vi "OE1022_Configure DAC.vi"(7 "OE1022_Configure DAC":T1 {"DAC4 Output" min=-10.0 max=10.0 format="%#_4g"; "DAC3 Output" min=-10.0 max=10.0 format="%#_4g"; "DAC2 Output" min=-10.0 max=10.0 format="%#_4g"; "DAC1 Output" min=-10.0 max=10.0 format="%#_4g"}, 8 "Error in (no error)":errorcluster caption="error out（no error）", 9 "Remote Mode":u16(ring) items=["USB"=0, "GPIB"=2], 11 "VISA resource name":refnum<visa-resource-name>) -> (0 "Error out":errorcluster caption="error out", 1 "Output String":string, 3 "VISA resource  out":refnum<visa-resource-name>)   [LabVIEW 2011]
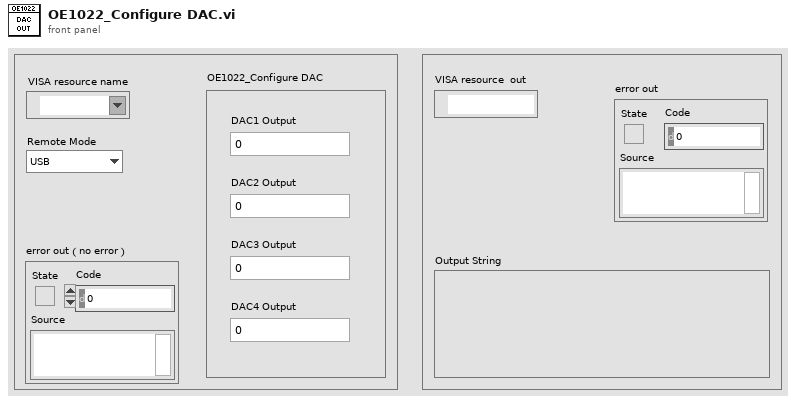
[diagram p1: front panel]
types:
  T1 = cluster{"DAC1 Output":dbl, "DAC2 Output":dbl, "DAC3 Output":dbl, "DAC4 Output":dbl}
  T2 = enum16{"ISRC", "IGND", "ICPL", "ILIN", "PHAS", "FMOD", "RSLP", "FREQ", "SWPT", "SLLM", "SULM", "SSLL", "SSLG", "STLM", "SWRM", "IRNG", "SENS", "RMOD", "OFLT", "OFSL", "SYNC", "DMOD", "HARM", "DARB", "SWVT", "SLVL", "SVLL", "SVUL", "SVSL", "SVSG", "SVTM", "SVRM", "RALL", "SNAP", "OUTP", "OAUX", "COUT", "CAUX", "COFP", "CEXP", "FPOP", "OEXP", "*IDN", "*RST", "OVLD", "INOV", "GNOV", "*PLL", "SSET", "RSET", "AGAN", "APHS", "ARSV", "ASCL", "EQCD", "EQCS", "SPED", "SRAT", "SLEN", "SSLE", "STRG", "SPRM", "STRD", "PAUS", "REST", "SPTS", "TRCA", "TEMP", "RSTU", "IHNZ", "DEQU", "SADD", "ARNG", "CSPE", "ISRCD", "IGNDD", "ICPLD", "ILIND", "PHASD", "FMODD", "RSLPD", "FREQD", "SWPTD", "SLLMD", "SULMD", "SSLLD", "SSLGD", "STLMD", "SWRMD", "SENSD", "RMODD", "OFLTD", "OFSLD", "SYNCD", "HARMD", "EQCDD", "EQCSD", "SNAPD", "OUTPD", "SWVTD", "SLVLD", "SVLLD", "SVULD", "SVSLD", "SVSGD", "SVTMD", "SVRMD", "SVDCD", "ARSVD", "AGAND", "APHSD", "ASCLD", "FPOPD", "CAUXD", "OEXPD", "SPEDD", "SRATD", "SLEND", "SSLED", "STRGD", "SPRMD", "STRDD", "PAUSD", "RESTD", "SPTSD", "TRCAD", "*IDND", "*RSTD", "INOVD", "GNOVD", "*PLLD", "SSETD", "RSETD"}
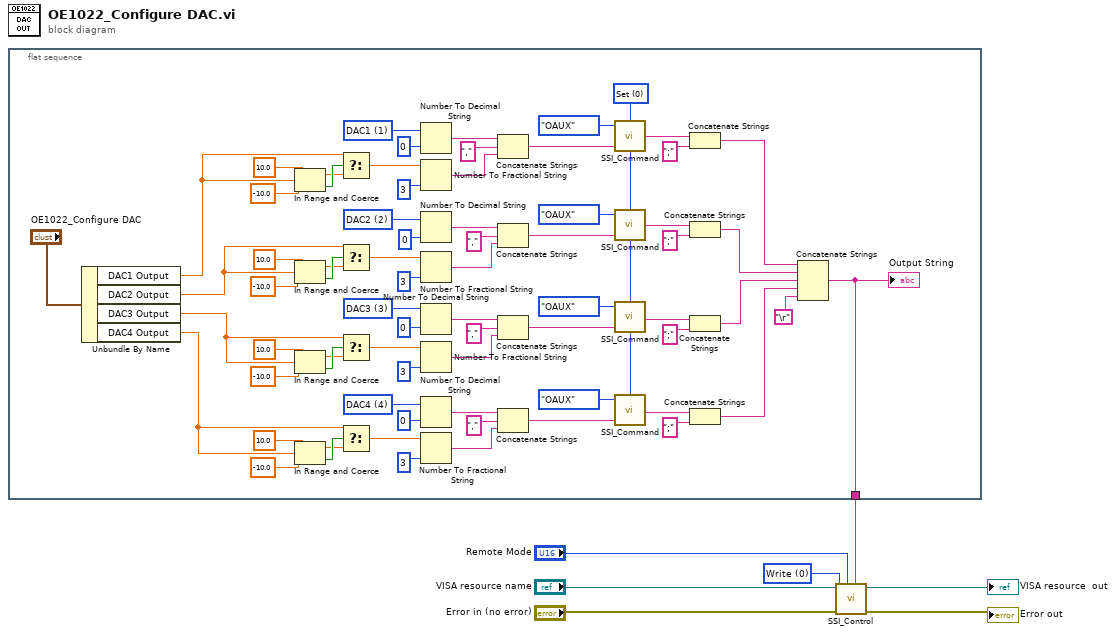
[diagram p0: block diagram]
diagram:
  w6 = u16 0 items=["Write", "Read"] ("Control")
  n1 = flat-sequence {
    tunnel: [w70] -> w1
    frame #0 {
      w8 = u16 0 items=["Set", "Query"] ("Opera")
      w9 = u16 4 items=["DAC1"=1, "DAC2"=2, "DAC3"=3, "DAC4"=4]
      w10 = u16 3 items=["DAC1"=1, "DAC2"=2, "DAC3"=3, "DAC4"=4]
      w11 = u16 2 items=["DAC1"=1, "DAC2"=2, "DAC3"=3, "DAC4"=4]
      w12 = u16 1 items=["DAC1"=1, "DAC2"=2, "DAC3"=3, "DAC4"=4]
      n2 = Unbundle By Name("OE1022_Configure DAC") -> ("DAC1 Output"=w44:dbl, "DAC2 Output"=w45:dbl, "DAC3 Output"=w46:dbl, "DAC4 Output"=w43:dbl)
      n3 = In Range and Coerce(upper limit=10.0 ("上限"), x=w44, lower limit=-10.0 ("下限")) -> (coerced(x)=w56:dbl, In Range?=w57:bool)
      n4 = In Range and Coerce(upper limit=10.0 ("上限"), x=w45, lower limit=-10.0 ("下限")) -> (coerced(x)=w63:dbl, In Range?=w64:bool)
      n5 = In Range and Coerce(upper limit=10.0 ("上限"), x=w46, lower limit=-10.0 ("下限")) -> (coerced(x)=w76:dbl, In Range?=w77:bool)
      n6 = In Range and Coerce(upper limit=10.0 ("上限"), x=w43, lower limit=-10.0 ("下限")) -> (coerced(x)=w60:dbl, In Range?=w61:bool)
      n7 = Select(t=w44, s=w57, f=w56) -> (s? t:f=w17:dbl)
      n8 = Select(t=w45, s=w64, f=w63) -> (s? t:f=w14:dbl)
      n9 = Select(t=w46, s=w77, f=w76) -> (s? t:f=w15:dbl)
      n10 = Select(t=w43, s=w61, f=w60) -> (s? t:f=w16:dbl)
      n11 = Number To Decimal String(number=w12, width (-)=i16 0 ("精度(6)")) -> (decimal integer string=w37:string)
      n12 = Number To Fractional String(number=w17, precision (6)=i16 3 ("宽度(-)")) -> (F-format string=w36:string)  [unwired: 2 in]
      n13 = Number To Decimal String(number=w11, width (-)=i16 0 ("宽度(-)")) -> (decimal integer string=w31:string)
      n14 = Number To Fractional String(number=w14, precision (6)=i16 3 ("宽度(-)")) -> (F-format string=w30:string)  [unwired: 2 in]
      n15 = Number To Decimal String(number=w10, width (-)=i16 0 ("精度(6)")) -> (decimal integer string=w29:string)
      n16 = Number To Fractional String(number=w15, precision (6)=i16 3 ("宽度(-)")) -> (F-format string=w28:string)  [unwired: 2 in]
      n17 = Number To Decimal String(number=w9, width (-)=i16 0 ("精度(6)")) -> (decimal integer string=w27:string)
      n18 = Number To Fractional String(number=w16, precision (6)=i16 3 ("宽度(-)")) -> (F-format string=w26:string)  [unwired: 2 in]
      n19 = Concatenate Strings(w37, "," ("替换字符串(\"\")"), w36) -> (w35:string)
      n20 = Concatenate Strings(w31, "," ("替换字符串(\"\")"), w30) -> (w25:string)
      n21 = Concatenate Strings(w29, "," ("替换字符串(\"\")"), w28) -> (w24:string)
      n22 = Concatenate Strings(w27, "," ("替换字符串(\"\")"), w26) -> (w23:string)
      n23 = call "SSI_Command.vi"("Opera"=w8, "Paramter"=w35, "Command Type"=T2."OAUX") -> ("Output string"=w47:string)  [unwired: 1 in]
      n24 = call "SSI_Command.vi"("Opera"=w8, "Paramter"=w25, "Command Type"=T2."OAUX") -> ("Output string"=w72:string)  [unwired: 1 in]
      n25 = call "SSI_Command.vi"("Opera"=w8, "Paramter"=w24, "Command Type"=T2."OAUX") -> ("Output string"=w65:string)  [unwired: 1 in]
      n26 = call "SSI_Command.vi"("Opera"=w8, "Paramter"=w23, "Command Type"=T2."OAUX") -> ("Output string"=w51:string)  [unwired: 1 in]
      n27 = Concatenate Strings(w47, ";" ("替换字符串(\"\")")) -> (w22:string)
      n28 = Concatenate Strings(w72, ";" ("替换字符串(\"\")")) -> (w21:string)
      n29 = Concatenate Strings(w65, ";" ("替换字符串(\"\")")) -> (w20:string)
      n30 = Concatenate Strings(w51, ";" ("替换字符串(\"\")")) -> (w19:string)
      n31 = Concatenate Strings(w22, w21, w20, w19, "\r") -> (w70:string)
      "Output String" <- w70
    }
  }
  n32 = call "SSI_Control.vi"("Write Buffer"=w1, "Remote Mode"="Remote Mode", "Error in (no error)"="Error in (no error)", "Control"=w6, "VISA resource name"="VISA resource name") -> ("Error out"=→"Error out":errorcluster, "VISA resource  out"=→"VISA resource  out":refnum<visa-resource-name>)  [unwired: 3 in, 2 out]
